vi "autoExample.vi"(8 "error in (no error)":errorcluster) -> (0 "error out":errorcluster)   [LabVIEW 2015]
panel:
  # "Remember when adding errors to the connector pane they go in the bottom 2"
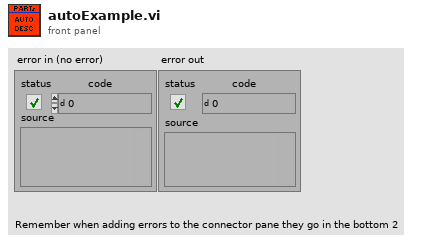
[diagram p1: front panel]
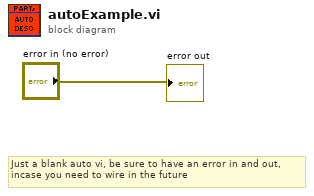
[diagram p0: block diagram]
diagram:
  # "Just a blank auto vi, be sure to have an error in and out, \nincase you need to wire in the future"
  "error out" <- "error in (no error)"
